vi "TxPkt - Is Buffered Transmit.vi"(8 "error in (no error)":errorcluster, 11 "Node Ptr In":T2 format="%.0x") -> (0 "error out":errorcluster, 2 "Packet Type":T1, 3 "Node Ptr Out":T2 format="%.0x")   [LabVIEW 2016, in "UDP-Custom-Device System Explorer.lvlib"]
uses:
  UDP-Custom-Device System Explorer.lvlib
  <vilib>/NI Veristand/Custom Device API/Custom Device Item Ref.ctl
  Types/Packet Info/Packet Type.ctl
  Shared/Constants.vi
  Shared/UDP-Custom-Device Shared.lvlib
  <vilib>/NI VeriStand/Custom Device API/Custom Device API.lvlib
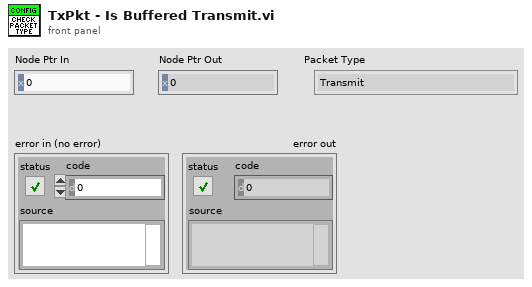
[diagram p1: front panel]
types:
  T1 = typedef "UDP-Custom-Device System Explorer.lvlib/Packet Type.ctl" = enum16{"Transmit", "Receive", "Buffered Transmit", "Buffered Receive"}
  T2 = typedef "Custom Device API.lvlib/Custom Device Item Ref.ctl" = u64
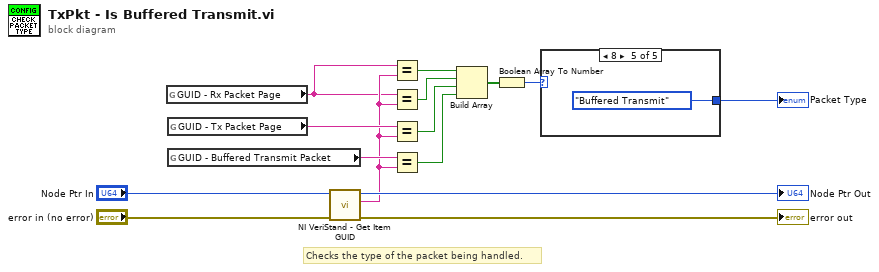
[diagram p0: block diagram]
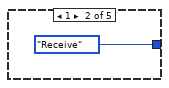
[diagram p3: hidden frame]
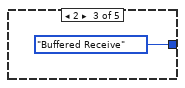
[diagram p4: hidden frame]
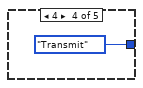
[diagram p5: hidden frame]
diagram:
  # "Checks the type of the packet being handled."
  n1 = global read "Constants.vi" "GUID - Rx Packet Page"() -> (w1:string)
  n2 = global read "Constants.vi" "GUID - Tx Packet Page"() -> (w3:string)
  n3 = global read "Constants.vi" "GUID - Buffered Transmit Packet"() -> (w4:string)
  n4 = call <vilib>:"NI VeriStand - Get Item GUID.vi"("error in (no error)"="error in (no error)", "Item Ref in"="Node Ptr In") -> ("error out"=→"error out":errorcluster, "GUID"=w2:string, "Item Ref out"=→"Node Ptr Out":T2)  [unwired: 7 in]
  n5 = Equal?(x=w1, y=w2) -> (x = y?=w11:bool)
  n6 = Equal?(x=w1, y=w2) -> (x = y?=w10:bool)
  n7 = Equal?(x=w3, y=w2) -> (x = y?=w9:bool)
  n8 = Equal?(x=w4, y=w2) -> (x = y?=w8:bool)
  n9 = Build Array(w11, w10, w9, w8) -> (w7:bool[])
  n10 = Boolean Array To Number(Boolean array=w7) -> (number=w6:u32)
  n11 = case shown="8" w6 {
    tunnel: [_ Packet_Type."Receive" ("Packet Type") Packet_Type."Buffered Receive" ("Packet Type") Packet_Type."Transmit" ("Packet Type") Packet_Type."Buffered Transmit" ("Packet Type")] -> w5
    frame 0, Default {
    }
    frame 1 {
    }
    frame 2 {
    }
    frame 4 {
    }
    frame 8 {
    }
  }
  "Packet Type" <- w5
